vi "Time 2 Record.vi"(1 "Step":string, 2 "Time Stamp":timestamp) -> (0 "String":string)   [LabVIEW 2009]
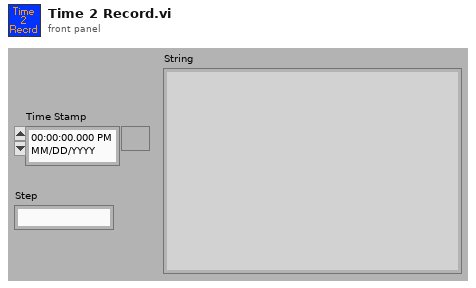
[diagram p1: front panel]
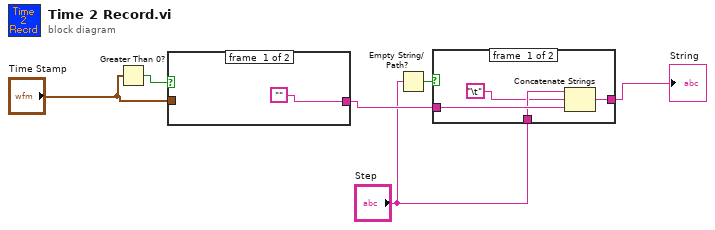
[diagram p0: block diagram]
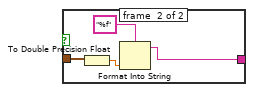
[diagram p3: hidden frame]
diagram:
  n1 = Greater Than 0?(x="Time Stamp") -> (x > 0?=w1:bool)
  n2 = case shown="True" w1 {
    tunnel: "Time Stamp" -> [_ w9]
    tunnel: ["" w8] -> w6
    frame #0 {
    }
    frame #1 {
      n3 = To Double Precision Float(number=w9) -> (double precision float=w10:dbl)
      n4 = Format Into String(format string="%f", w10) -> (resulting string=w8:string)  [unwired: 2 in, 1 out]
    }
  }
  n5 = Empty String/Path?(string/path="Step") -> (empty?=w4:bool)
  n6 = case shown="False" w4 {
    tunnel: [w15 w16] -> w3
    tunnel: "Step" -> [w13 _]
    tunnel: w6 -> [w14 w16]
    frame #0 {
      n7 = Concatenate Strings(w13, "\t", w14) -> (w15:string)
    }
    frame #1 {
    }
  }
  "String" <- w3
